vi "Get All Items From Enumerator.vi"(8 "error in (no error)":errorcluster caption="错误输入（无错误）", 11 "Enumerator 输入":refnum<class "Enumerator.lvclass"> caption="DNL_LabVIEW Object in") -> (0 "error out":errorcluster caption="错误输出", 2 "Items":variant[](array[variant]), 3 "Enumerator 输出":refnum<class "Enumerator.lvclass"> caption="DNL_LabVIEW Object out")   [LabVIEW 2012, in "Enumerator.lvclass"]
uses:
  Enumerator.lvclass
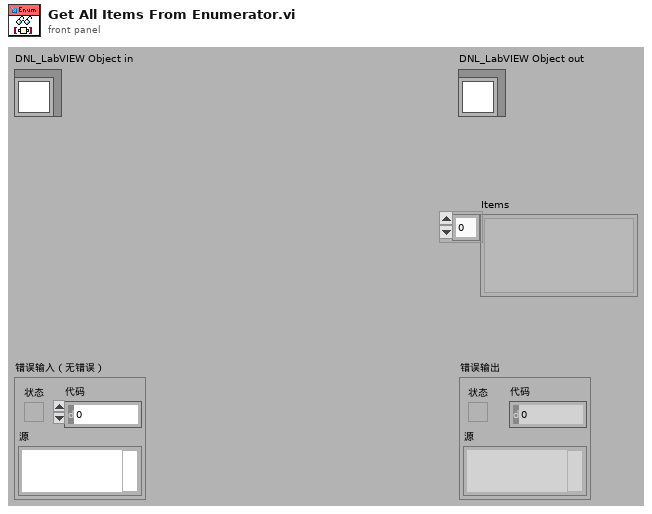
[diagram p1: front panel]
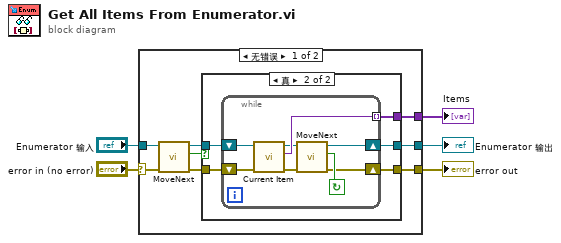
[diagram p0: block diagram]
diagram:
  n1 = case shown="无错误" "error in (no error)" {
    selector: "error in (no error)" -> [w12 w30]
    tunnel: [w6 w30] -> w4
    tunnel: [w7 w29] -> w2
    tunnel: "Enumerator 输入" -> [w13 w29]
    tunnel: [w8 _] -> w1
    frame No Error {
      n2 = call "MoveNext.vi"("error in (no error)"=w12, "Enumerator 输入"=w13) -> ("error out"=w9:errorcluster, "MoveNext"=w11:bool, "Enumerator 输出"=w10:refnum<class "Enumerator.lvclass">)  [unwired: 7 in]
      n3 = case shown="真" w11 {
        tunnel: w10 -> [w14 w20]
        tunnel: w9 -> [w15 w19]
        tunnel: [_ w18] -> w8
        tunnel: [w14 w17] -> w7
        tunnel: [w15 w16] -> w6
        frame False {
        }
        frame True {
          n4 = while {
            shift-right: [w21] -> w17
            shift-left: w20 -> [w28]
            shift-right: [w22] -> w16
            shift-left: w19 -> [w27]
            tunnel: [w26] -> w18 mode=indexing
            stop <- w23 continue-if-true
            n5 = call "Current Item.vi"("error in (no error)"=w27, "Enumerator 输入"=w28) -> ("error out"=w25:errorcluster, "Item"=w26:variant, "Enumerator 输出"=w24:refnum<class "Enumerator.lvclass">)  [unwired: 7 in]
            n6 = call "MoveNext.vi"("error in (no error)"=w25, "Enumerator 输入"=w24) -> ("error out"=w22:errorcluster, "MoveNext"=w23:bool, "Enumerator 输出"=w21:refnum<class "Enumerator.lvclass">)  [unwired: 7 in]
          }
        }
      }
    }
    frame Error {
    }
  }
  "error out" <- w4
  "Enumerator 输出" <- w2
  "Items" <- w1
